vi "stringToUTF8Array.vi"(7 "string":string) -> (8 "UTF8[]":u8[](array[numeric]))   [LabVIEW 2018]
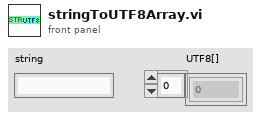
[diagram p1: front panel]
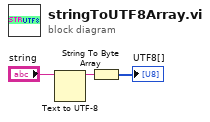
[diagram p0: block diagram]
diagram:
  n1 = Text to UTF-8(11:"string") -> (3:w2:string)  [unwired: 2 in, 1 out]
  n2 = String To Byte Array(string=w2) -> (unsigned byte array=→"UTF8[]":u8[])
